vi "Initialize.vi"(0 "Program List From SFTP in":refnum<class "Program List From SFTP.lvclass">, 5 "error in (no error)":errorcluster, 8 "Application.lvclass":refnum<class "Application.lvclass">) -> (14 "Program List From SFTP out":refnum<class "Program List From SFTP.lvclass">, 19 "error out":errorcluster)   [LabVIEW 2019, in "Program List From SFTP.lvclass"]
uses:
  Program List From SFTP.lvclass
  Application.lvclass
  Program List From SFTP.lvclass/Program List From SFTP.ctl
  LabSSH Library/SFTP Library/Connection Info..cluster.ctl
  LabSSH Library/SFTP Library/Password..cluster.ctl
  LabSSH Library/SFTP Library/connect_password.vi
  Program List/Program List.lvclass
  LabSSH Library/SFTP Library/LabSFTP.lvlib
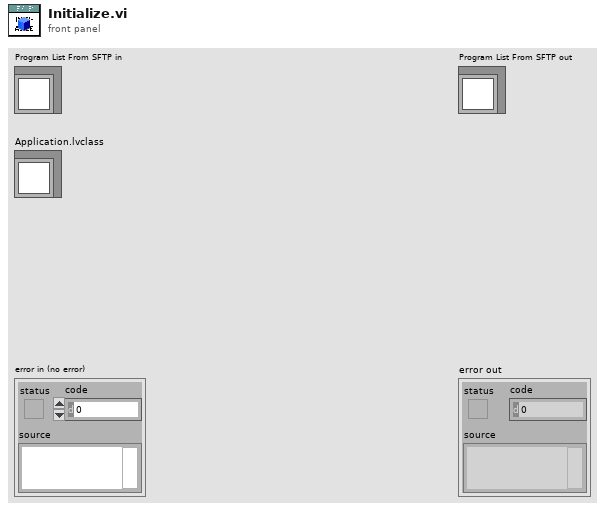
[diagram p1: front panel]
types:
  T1 = typedef "LabSFTP.lvlib/Password..cluster.ctl" = cluster{"Password":string}
  T2 = typedef "LabSFTP.lvlib/Connection Info..cluster.ctl" = cluster{"Remote":string, "Username":string, "Port (22)":i32}
  T3 = typedef "Application.lvclass/ApplicationSettings.ctl" = cluster{"Robot IP":string, "Socket Host IP":string, "Robot Type":T4, "Use SFTP Program List":bool, "Robot Logging":bool, "TCP Logging":bool, "Fault Program":string}
  T4 = typedef "Application.lvclass/RobotType.ctl" = enum16{"UR E-Series", "UR CB-Series"}
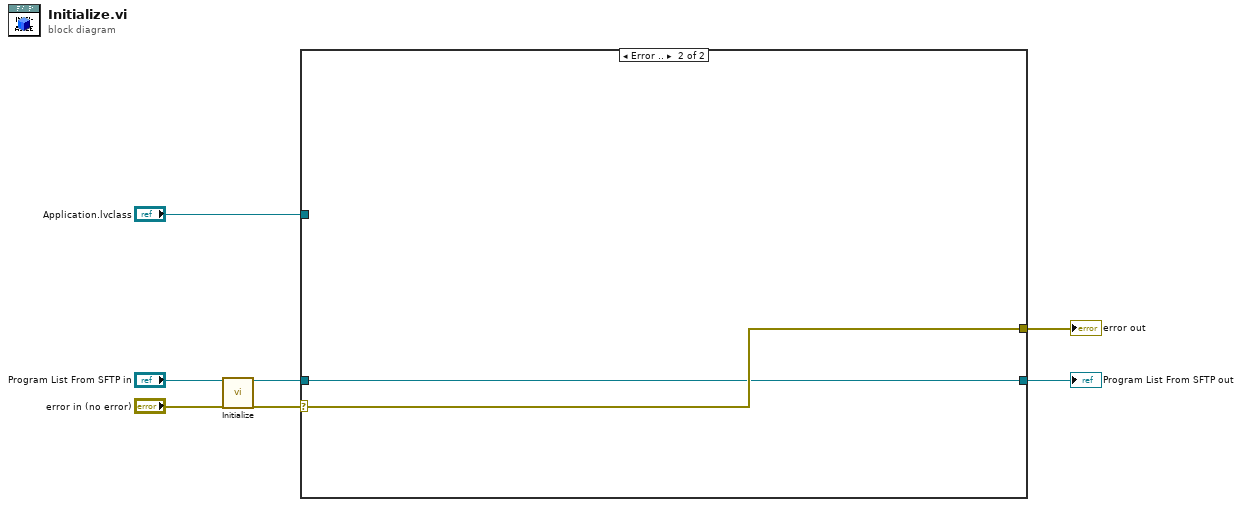
[diagram p0: block diagram]
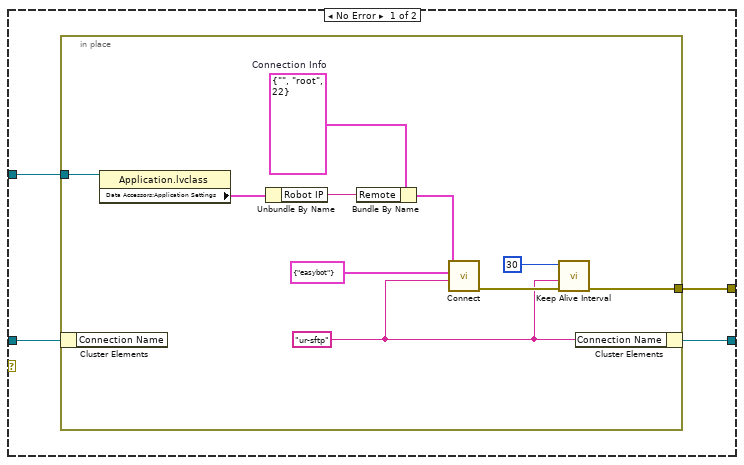
[diagram p2: hidden frame]
diagram:
  n1 = call-parent "Initialize.vi"("Program List in"="Program List From SFTP in", "error in (no error)"="error in (no error)") -> ("Program List out"=w3:refnum<class "Program List From SFTP.lvclass">, "error out"=w2:errorcluster)  [unwired: 16 in]
  n2 = case shown="Error .." w2 {
    selector: w2 -> [_ w23]
    tunnel: [w11 w23] -> w7
    tunnel: "Application.lvclass" -> [w10 _]
    tunnel: w3 -> [w9 w22]
    tunnel: [w8 w22] -> w1
    frame No Error {
      n3 = in-place {
        in-place-border: [w16] -> w11
        in-place-border: w10 -> [w15]
        w12 = "ur-sftp" ("Connection Name")
        w18 = T2 {"Remote"="", "Username"="root", "Port (22)"=22}  # Connection Info
        n4 = in-place-cluster #1(w9) -> ()  [unwired: 1 out]
        n5 = property class="Application.lvclass"(reference=w15) -> ("Data Accessors:Application Settings"=w14:T3)  [unwired: 1 in, 2 out]
        n6 = Unbundle By Name(w14) -> ("Robot IP"=w13:string)
        n7 = Bundle By Name(cluster=w18, "Remote"=w13) -> (w17:T2)
        n8 = call-poly "Connect.vi"("Connection Name"=w12, "Password"=T1 {"Password"="easybot"}, "Connection Info."=w17) -> ("error out"=w19:errorcluster)  [unwired: 6 in, 2 out]
        n9 = call "Keep Alive Interval.vi"("error in (no error)"=w19, "Connection Name"=w12, "Keep Alive Interval (s)"=30) -> ("error out"=w16:errorcluster)  [unwired: 8 in]
        n10 = in-place-cluster #1("Connection Name"=w12) -> (w8:refnum<class "Program List From SFTP.lvclass">)
      }
    }
    frame Error {
    }
  }
  "error out" <- w7
  "Program List From SFTP out" <- w1
